vi "Number of CPUs Dialog.vi"(8 "error in (no error)":errorcluster) -> (0 "error out":errorcluster, 3 "CPU_Cores":i32=4 min=1 step=1)   [LabVIEW 2011, in "System Monitor Custom Device.lvlib"]
uses:
  System Monitor Custom Device.lvlib
panel:
  in  "OK":bool
  in  "CPU Cores":i32=4 min=1 step=1
  # "How many CPU cores do you wish to monitor?"
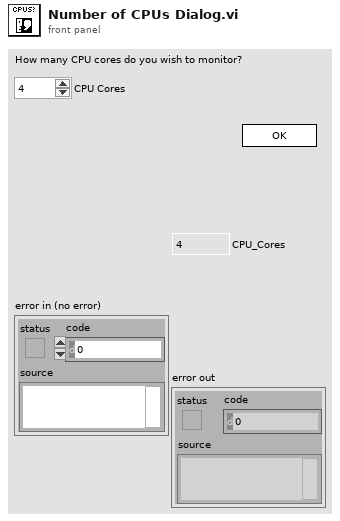
[diagram p1: front panel]
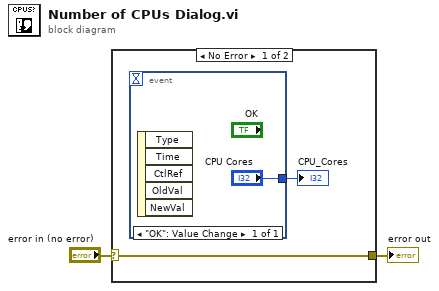
[diagram p0: block diagram]
diagram:
  n1 = case shown="No Error" "error in (no error)" {
    selector: "error in (no error)" -> [w3 w6]
    tunnel: [w3 w6] -> w1
    frame No Error {
      n2 = event shown="[0] \"OK\": Value Change" {
        selector: _ -> [_]
        dyn-events: _ -> [_]
        timeout: _ -> [_]
        tunnel: ["CPU Cores"] -> w4
        event "OK": Value Change {
          n3 = event-data() -> ()  [unwired: 1 in, 5 out]
        }
      }
      "CPU_Cores" <- w4
    }
    frame Error {
    }
  }
  "error out" <- w1
